vi "TransSpeed.vi"(1 "Speed_In":i32) -> (0 "Speed_Out":i32)   [LabVIEW 2011]
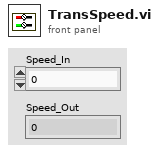
[diagram p1: front panel]
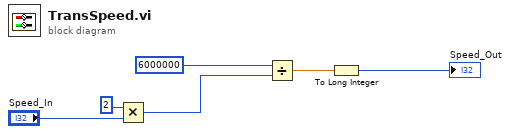
[diagram p0: block diagram]
diagram:
  n1 = Multiply(x=2, y="Speed_In") -> (x*y=w3:i32)
  n2 = Divide(x=6000000, y=w3) -> (x/y=w2:dbl)
  n3 = To Long Integer(number=w2) -> (32bit integer=→"Speed_Out":i32)
